vi "Test Insert VI Into SubPanel.vi"(11 "Test Case In":refnum<class "Test Insert VI into SubPanel.lvclass">) -> (0 "error out":errorcluster, 3 "Test Case Out":refnum<class "Test Insert VI into SubPanel.lvclass">)   [LabVIEW 2024, in "Test Insert VI into SubPanel.lvclass"]
uses:
  Test Insert VI into SubPanel.lvclass
  C:/Program Files/National Instruments/LabVIEW 2025/vi.lib/Astemes/LUnit/Test Case.lvclass
  <vilib>/Astemes/LUnit/Test Case.lvclass/Test Case.ctl
  Test Insert VI into SubPanel.lvclass/Test Insert VI into SubPanel.ctl
  Source/Common Helpers.lvlib
  <vilib>/Astemes/LUnit/Test Case.lvclass
  C:/Program Files/National Instruments/LabVIEW 2025/vi.lib/Astemes/LUnit/LUnit Runnable.lvclass
  D:/git/Open-Xml-LabVIEW/Common-Labview-helpers/Test Insert VI into SubPanel/Test Insert VI into SubPanel.lvclass
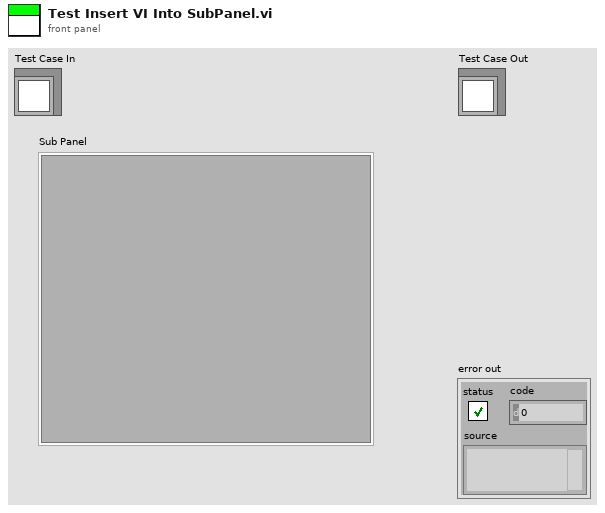
[diagram p1: front panel]
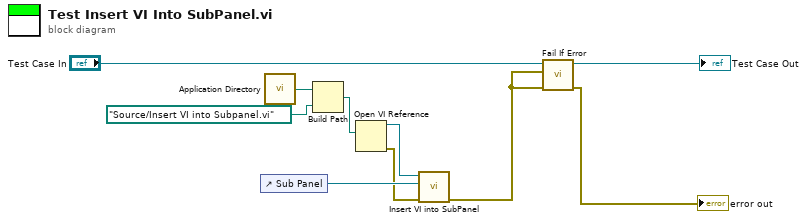
[diagram p0: block diagram]
diagram:
  n1 = control-ref of="Sub Panel"() -> (w7:refnum<vi>)
  n2 = call <vilib>:"Application Directory.vi"() -> ("Application Directory"=w5:path)
  n3 = Build Path(base path=w5, name or relative path=path "Source/Insert VI into Subpanel.vi") -> (appended path=w3:path)
  n4 = Open VI Reference(vi path=w3) -> (vi reference=w2:refnum<vi>, error out=w1:errorcluster)  [unwired: 5 in]
  n5 = call "Insert VI into SubPanel.vi"("error in"=w1, "SubPnl Ref"=w7, "VI Ref"=w2) -> ("error out"=w6:errorcluster)  [unwired: 8 in]
  n6 = call <vilib>:"Fail If Error.vi"("error in (no error)"=w6, "Assert error"=w6, "LUnit Test Case In"="Test Case In") -> ("error out"=→"error out":errorcluster, "LUnit Test Case Out"=→"Test Case Out":refnum<class "Test Insert VI into SubPanel.lvclass">)  [unwired: 7 in]
